vi "HIZ STOP.vi"(0 "class data in":refnum<class "MB_ENGINE.lvclass">, 11 "error in (no error)":errorcluster) -> (4 "class data out":refnum<class "MB_ENGINE.lvclass">, 15 "error out":errorcluster)   [LabVIEW 2019, in "MB_ENGINE.lvclass"]
uses:
  MB_ENGINE.lvclass
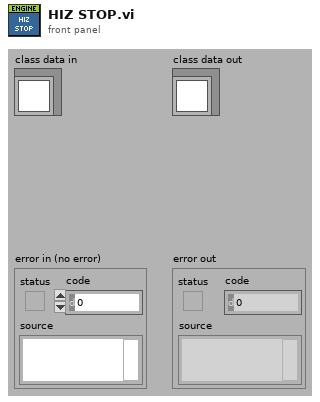
[diagram p1: front panel]
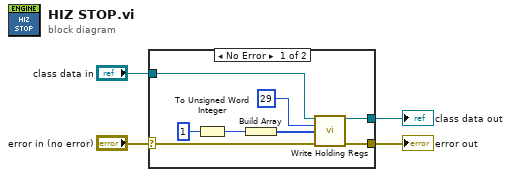
[diagram p0: block diagram]
diagram:
  n1 = case shown="No Error" "error in (no error)" {
    selector: "error in (no error)" -> [w10 w14]
    tunnel: [w9 w14] -> w3
    tunnel: "class data in" -> [w12 w13]
    tunnel: [w5 w13] -> w1
    frame No Error {
      n2 = To Unsigned Word Integer(number=u16 1) -> (unsigned 16bit integer=w8:u16)
      n3 = Build Array(w8) -> (w7:u16[])
      n4 = call-dynamic "Write Holding Regs.vi"("reference in"=w12, "starting address"=u16 29, "Regs"=w7, "error in (no error)"=w10) -> ("reference out"=w5:refnum<class "MB_ENGINE.lvclass">, "error out"=w9:errorcluster)  [unwired: 10 in]
    }
    frame Error {
    }
  }
  "error out" <- w3
  "class data out" <- w1
